vi "LED Control.vi"   [LabVIEW 2012]
uses:
  <vilib>/Rock Robotics/WPI/Relay/WPI_RelayValue.ctl
  Globals/Jaguar Commands.vi
  Globals/Shooter Speed Error.vi
types:
  T1 = typedef "WPI_RelayDevRef.ctl" = cluster{"DevStatus":errorcluster, "Relay Channel":T2, "Digital Module":T3, "Relay Direction":T4}
  T2 = typedef "FPGA_DIORelayChannel.ctl" = enum8{"Relay 1", "Relay 2", "Relay 3", "Relay 4", "Relay 5", "Relay 6", "Relay 7", "Relay 8", "Invalid"}
  T3 = typedef "FPGA_TypedefDigitalModule.ctl" = enum16{"Digital Module 1", "Digital Module 2"}
  T4 = typedef "WPI_RelayDirection.ctl" = enum16{"Both directions", "Forward only", "Reverse only"}
  T5 = typedef "WPI_RelayValue.ctl" = enum16{"Off", "On", "Forward", "Reverse"}
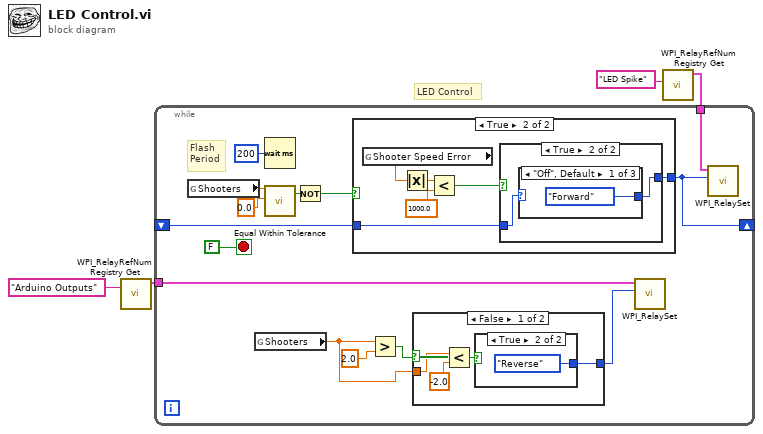
[diagram p0: block diagram]
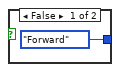
[diagram p2: hidden frame]
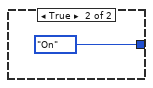
[diagram p3: hidden frame]
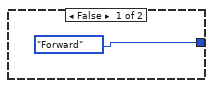
[diagram p4: hidden frame]
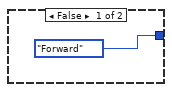
[diagram p5: hidden frame]
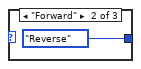
[diagram p6: hidden frame]
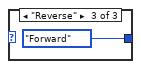
[diagram p7: hidden frame]
diagram:
  # "LED Control"
  n1 = call <vilib>:"WPI_RelayRefNum Registry Get.vi"("refnum name"="Arduino Outputs") -> ("RelayDevRef"=w1:T1)  [unwired: 9 in, 1 out]
  n2 = call <vilib>:"WPI_RelayRefNum Registry Get.vi"("refnum name"="LED Spike") -> ("RelayDevRef"=w3:T1)  [unwired: 9 in, 1 out]
  n3 = while {
    tunnel: w3 -> [w10]
    shift-right: [w15] -> _
    shift-left: _ -> [w14]
    tunnel: w1 -> [w9]
    stop <- FALSE stop-if-true
    # "Flash\nPeriod"
    n4 = global read "Jaguar Commands.vi" "Shooters"() -> (w18:dbl)
    n5 = global read "Jaguar Commands.vi" "Shooters"() -> (w5:dbl)
    n6 = Wait (ms)(milliseconds to wait=u32 200) -> ()  [unwired: 1 out]
    n7 = call "Equal Within Tolerance.vi"("Number In"=w18, "Comparison Value"=0.0) -> ("Equality"=w16:bool)  [unwired: 17 in]
    n8 = Not(x=w16) -> (.not. x?=w11:bool)
    n9 = case shown="True" w11 {
      tunnel: [WPI_RelayValue."Forward" ("RelayValue") w28] -> w15
      tunnel: w14 -> [_ w27]
      frame False {
      }
      frame True {
        n10 = global read "Shooter Speed Error.vi" "Shooter Speed Error"() -> (w32:dbl)
        n11 = Absolute Value(x=w32) -> (abs(x)=w30:dbl)
        n12 = Less?(x=w30, y=1000.0) -> (x < y?=w29:bool)
        n13 = case shown="True" w29 {
          tunnel: [WPI_RelayValue."Forward" ("RelayValue") w34] -> w28
          tunnel: w27 -> [_ w35]
          frame False {
          }
          frame True {
            n14 = case shown="\"Off\", Default" w35 {
              tunnel: [WPI_RelayValue."Forward" ("RelayValue") WPI_RelayValue."Reverse" ("RelayValue") WPI_RelayValue."Forward" ("RelayValue")] -> w34
              frame "Off", Default {
              }
              frame "Forward" {
              }
              frame "Reverse" {
              }
            }
          }
        }
      }
    }
    n15 = Greater?(x=w5, y=2.0) -> (0:w6:bool)
    n16 = case shown="False" w6 {
      tunnel: [w22 WPI_RelayValue."On" ("RelayValue")] -> w8
      tunnel: w5 -> [w19 _]
      frame False {
        n17 = Less?(x=w19, y=-2.0) -> (x < y?=w21:bool)
        n18 = case shown="True" w21 {
          tunnel: [WPI_RelayValue."Forward" ("RelayValue") WPI_RelayValue."Reverse" ("RelayValue")] -> w22
          frame False {
          }
          frame True {
          }
        }
      }
      frame True {
      }
    }
    n19 = call <vilib>:"WPI_RelaySet.vi"("RelayValue"=w8, "RelayDevRef"=w9) -> ()  [unwired: 8 in, 2 out]
    n20 = call <vilib>:"WPI_RelaySet.vi"("RelayValue"=w15, "RelayDevRef"=w10) -> ()  [unwired: 8 in, 2 out]
  }
